vi "AutoApproach_FBL.vi"() -> ()   [LabVIEW 2019]
doc: "Programming Interface Example: Automatic approach implemented using Nanonis Programming Interface functions. This can be used if you want to execute special functions after each motor step or if you want to control your motor directly from LabVIEW.\n\n- Nanonis Programming Interface -"
uses:
  <userlib>/Nanonis Prog Interface V5/Nanonis Prog Interface.lvlib
  GlobalClicksHeight_FBL.vi
panel:
  out "Surface reached":bool
  in  "Wait for motor (ms)":u32=1000
  in  "Motor steps":u16=1
  in  "stop":bool
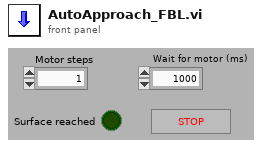
[diagram p1: front panel]
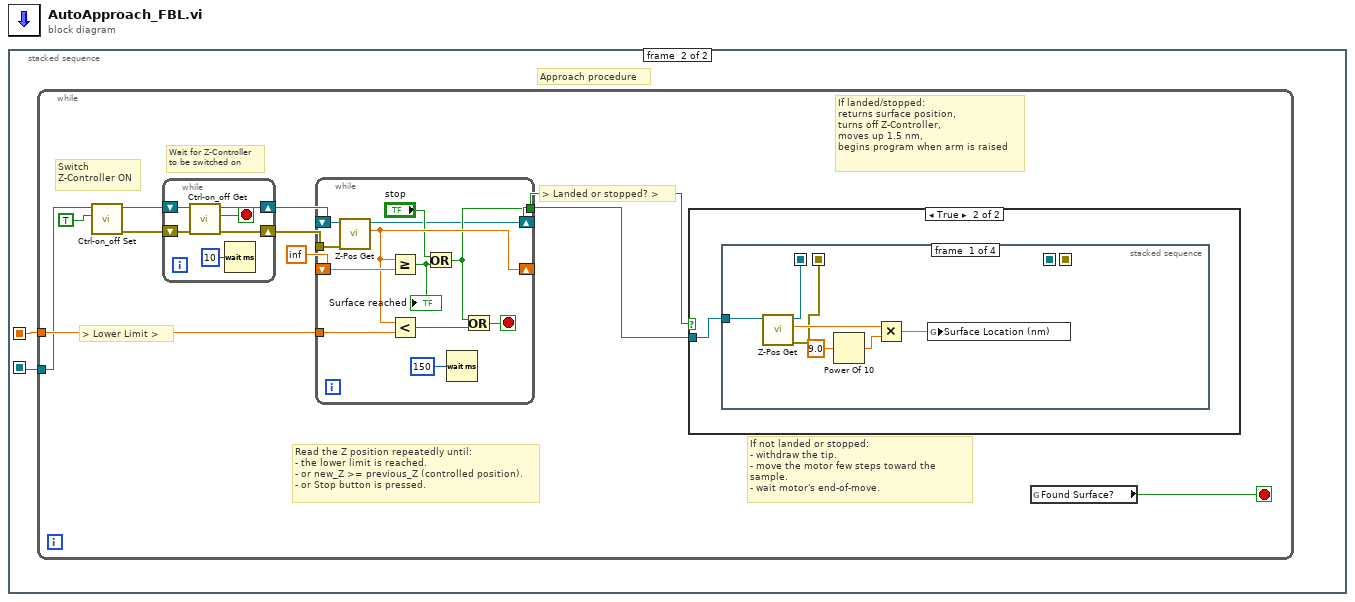
[diagram p0: block diagram]
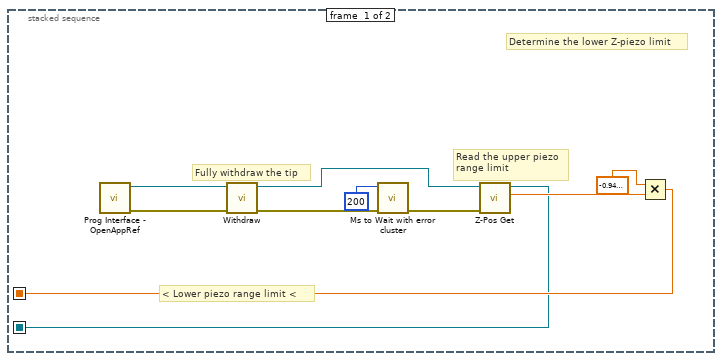
[diagram p2: hidden frame]
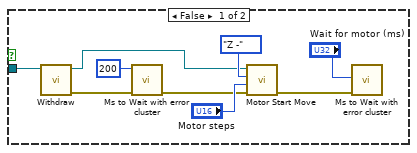
[diagram p3: hidden frame]
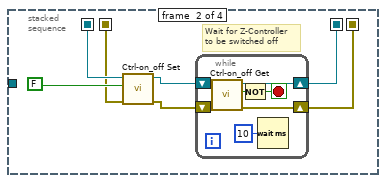
[diagram p4: hidden frame]
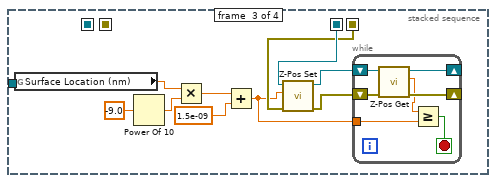
[diagram p5: hidden frame]
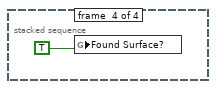
[diagram p6: hidden frame]
diagram:
  n1 = stacked-sequence {
    seq-local: [w9 _] -> [_ w12]
    seq-local: [w2 _] -> [_ w11]
    frame #0 {
      # "Read the upper piezo\nrange limit"
      # "Fully withdraw the tip"
      # "< Lower piezo range limit <"
      # "Determine the lower Z-piezo limit"
      n2 = call <userlib>:"Prog Interface - OpenAppRef.vi"() -> ("Error out"=w8:errorcluster, "Application reference"=w3:refnum<vi>)  [unwired: 6 in]
      n3 = call <userlib>:"Withdraw.vi"("Error in (no error)"=w8, "Application ref in"=w3) -> ("Error out"=w5:errorcluster, "Application ref out"=w1:refnum<vi>)  [unwired: 8 in]
      n4 = call <userlib>:"Ms to Wait with error cluster.vi"("error in (no error)"=w5, "milliseconds to wait"=u32 200) -> ("error out"=w4:errorcluster)  [unwired: 4 in, 1 out]
      n5 = call <userlib>:"Z-Pos Get.vi"("error in (no error)"=w4, "Application ref in"=w1) -> ("Z position (m)"=w7:sgl, "Application ref out"=w2:refnum<vi>)  [unwired: 7 in, 1 out]
      n6 = Multiply(x=sgl -0.95, y=w7) -> (x*y=w9:sgl)
    }
    frame #1 {
      # "Approach procedure"
      n7 = while {
        tunnel: w12 -> [w22]
        tunnel: w11 -> [w17]
        stop <- w13 stop-if-true
        # "If landed/stopped:  \nreturns surface position, \nturns off Z-Controller, \nmoves up 1.5 nm,\nbegins program when arm is raised"
        # "Wait for Z-Controller\nto be switched on"
        # "> Lower Limit >"
        # "Switch Z-Controller ON"
        # "> Landed or stopped? >"
        # "Read the Z position repeatedly until:\n- the lower limit is reached.\n- or new_Z >= previous_Z (controlled position).\n- or Stop button is pressed."
        # "If not landed or stopped:\n- withdraw the tip.\n- move the motor few steps toward the sample.\n- wait motor's end-of-move."
        n8 = call <userlib>:"Ctrl-on_off Set.vi"("Z Controller ON/OFF"=TRUE ("Ctrl on/off"), "Application ref in"=w17) -> ("error out"=w19:errorcluster, "Application ref out"=w16:refnum<vi>)  [unwired: 8 in]
        n9 = while {
          shift-right: [w29] -> w18
          shift-left: w19 -> [w28]
          shift-right: [w24] -> w15
          shift-left: w16 -> [w25]
          stop <- w27 stop-if-true
          n10 = call <userlib>:"Ctrl-on_off Get.vi"("error in (no error)"=w28, "Application ref in"=w25) -> ("error out"=w29:errorcluster, "Z-Controller on/off status"=w27:bool, "Application ref out"=w24:refnum<vi>)  [unwired: 7 in]
          n11 = Wait (ms)(milliseconds to wait=u32 10) -> ()  [unwired: 1 out]
        }
        n12 = while {
          shift-right: [w39] -> _
          shift-left: sgl inf ("Z-pos (m)") -> [w41]
          tunnel: [w35] -> w23
          tunnel: w22 -> [w33]
          tunnel: w18 -> [w32]
          shift-right: [w30] -> w14
          shift-left: w15 -> [w31]
          stop <- w36 stop-if-true
          n13 = call <userlib>:"Z-Pos Get.vi"("error in (no error)"=w32, "Application ref in"=w31) -> ("Z position (m)"=w39:sgl, "Application ref out"=w30:refnum<vi>)  [unwired: 7 in, 1 out]
          n14 = Greater Or Equal?(x=w39, y=w41) -> (x >= y?=w38:bool)
          "Surface reached" <- w38
          n15 = Less?(x=w39, y=w33) -> (x < y?=w37:bool)
          n16 = Or(x="stop", y=w38) -> (x .or. y?=w35:bool)
          n17 = Wait (ms)(milliseconds to wait=u32 150) -> ()  [unwired: 1 out]
          n18 = Or(x=w35, y=w37) -> (x .or. y?=w36:bool)
        }
        n19 = case shown="True" w23 {
          tunnel: w14 -> [w43 w51]
          frame False {
            n20 = call <userlib>:"Withdraw.vi"("Application ref in"=w43) -> ("Error out"=w48:errorcluster, "Application ref out"=w42:refnum<vi>)  [unwired: 9 in]
            n21 = call <userlib>:"Ms to Wait with error cluster.vi"("error in (no error)"=w48, "milliseconds to wait"=u32 200) -> ("error out"=w47:errorcluster)  [unwired: 4 in, 1 out]
            n22 = call <userlib>:"Motor Start Move.vi"("Error in (no error)"=w47, "Number of steps"="Motor steps", "Direction"=enum16{"X +", "X -", "Y +", "Y -", "Z +", "Z -"}."Z -", "Application ref in"=w42) -> ("Error out"=w45:errorcluster)  [unwired: 5 in, 1 out]
            n23 = call <userlib>:"Ms to Wait with error cluster.vi"("error in (no error)"=w45, "milliseconds to wait"="Wait for motor (ms)") -> ()  [unwired: 4 in, 2 out]
          }
          frame True {
            n24 = stacked-sequence {
              seq-local: [w54 _ _ _] -> [_ w64 _ _]
              seq-local: [w52 _ _ _] -> [_ w63 _ _]
              seq-local: [_ w60 _ _] -> [_ _ w77 _]
              seq-local: [_ w59 _ _] -> [_ _ w76 _]
              tunnel: w51 -> [w53 _ _ _]
              frame #0 {
                n25 = call <userlib>:"Z-Pos Get.vi"("Application ref in"=w53) -> ("error out"=w52:errorcluster, "Z position (m)"=w58:sgl, "Application ref out"=w54:refnum<vi>)  [unwired: 8 in]
                n26 = Power Of 10(x=9.0) -> (10^x=w57:dbl)
                n27 = Multiply(x=w58, y=w57) -> (x*y=w55:dbl)
                n28 = global write "GlobalClicksHeight_FBL.vi" "Surface Location (nm)"(w55) -> ()
              }
              frame #1 {
                # "Wait for Z-Controller\nto be switched off"
                n29 = call <userlib>:"Ctrl-on_off Set.vi"("error in (no error)"=w63, "Z Controller ON/OFF"=FALSE, "Application ref in"=w64) -> ("error out"=w61:errorcluster, "Application ref out"=w62:refnum<vi>)  [unwired: 7 in]
                n30 = while {
                  shift-right: [w72] -> w59
                  shift-left: w61 -> [w71]
                  shift-right: [w67] -> w60
                  shift-left: w62 -> [w68]
                  stop <- w66 stop-if-true
                  n31 = call <userlib>:"Ctrl-on_off Get.vi"("error in (no error)"=w71, "Application ref in"=w68) -> ("error out"=w72:errorcluster, "Z-Controller on/off status"=w70:bool, "Application ref out"=w67:refnum<vi>)  [unwired: 7 in]
                  n32 = Not(x=w70) -> (.not. x?=w66:bool)
                  n33 = Wait (ms)(milliseconds to wait=u32 10) -> ()  [unwired: 1 out]
                }
              }
              frame #2 {
                n34 = global read "GlobalClicksHeight_FBL.vi" "Surface Location (nm)"() -> (w80:dbl)
                n35 = Power Of 10(x=-9.0) -> (10^x=w82:dbl)
                n36 = Multiply(x=w80, y=w82) -> (x*y=w79:dbl)
                n37 = Add(x=w79, y=1.5e-09) -> (x+y=w73:dbl)
                n38 = call <userlib>:"Z-Pos Set.vi"("error in (no error)"=w76, "Z position (m)"=w73, "Application ref in"=w77) -> ("error out"=w74:errorcluster, "Application ref out"=w75:refnum<vi>)  [unwired: 7 in]
                n39 = while {
                  shift-right: [w86] -> _
                  shift-left: w74 -> [w88]
                  shift-right: [w87] -> _
                  shift-left: w75 -> [w89]
                  tunnel: w73 -> [w83]
                  stop <- w85 stop-if-true
                  n40 = call <userlib>:"Z-Pos Get.vi"("error in (no error)"=w88, "Application ref in"=w89) -> ("error out"=w86:errorcluster, "Z position (m)"=w84:sgl, "Application ref out"=w87:refnum<vi>)  [unwired: 7 in]
                  n41 = Greater Or Equal?(x=w84, y=w83) -> (x >= y?=w85:bool)
                }
              }
              frame #3 {
                n42 = global write "GlobalClicksHeight_FBL.vi" "Found Surface?"(TRUE ("Found Surface?")) -> ()
              }
            }
          }
        }
        n43 = global read "GlobalClicksHeight_FBL.vi" "Found Surface?"() -> (w13:bool)
      }
    }
  }
